vi "Get Created.vi"(11 "Base Addresses Strategy in":refnum<class "Base Addresses Strategy.lvclass">) -> (2 "Created":T1)   [LabVIEW 2021, in "jettl.lvlib" / "Addresses Strategy.lvlib" / "Base Addresses Strategy.lvclass"]
uses:
  Base Addresses Strategy.lvclass
  Created.ctl
  Msg/Msg.lvclass
  Base Addresses Strategy.lvclass/Base Addresses Strategy.ctl
  Addresses Strategy.lvlib
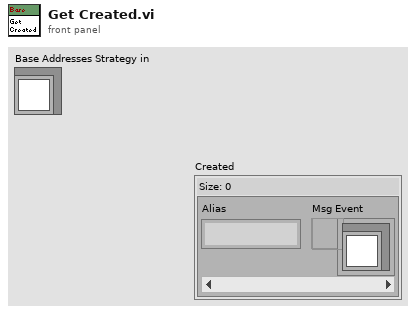
[diagram p1: front panel]
types:
  T1 = typedef "jettl.lvlib/Addresses Strategy.lvlib/Created.ctl" = map{string, refnum<user-event>}
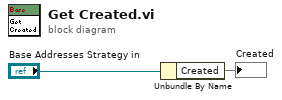
[diagram p0: block diagram]
diagram:
  n1 = Unbundle By Name("Base Addresses Strategy in") -> ("Created"=→"Created":T1)
